vi "IsArrayConstant__slk_mt.vi"(7 "create enum configure":T1, 8 "error in (no error)":errorcluster, 11 "selection list":refnum<vi>[](array[refnum])) -> (0 "error out":errorcluster, 2 "position":cluster{"Left":i32, "Top":i32}, 3 "values":string[](array[string]), 4 "not?":bool)   [LabVIEW 2010]
uses:
  TypeDef/TypeDef_CreateEnumConfigure__slk_mt.ctl
  Library/Lazyboots Menu Tool.lvlib
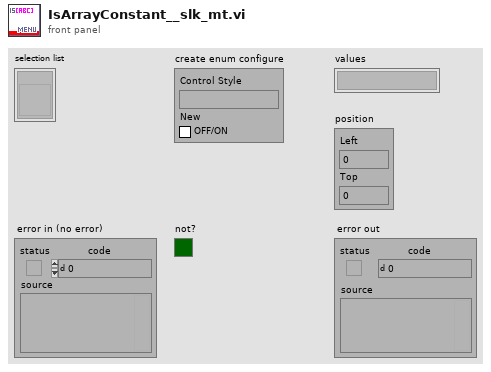
[diagram p1: front panel]
types:
  T1 = typedef "Lazyboots Menu Tool.lvlib/TypeDef_CreateEnumConfigure__slk_mt.ctl" = cluster{"Control Style":string, "New":bool}
  T2 = typedef "LVPositionTypeDef.ctl" = cluster{"Left":i32, "Top":i32}
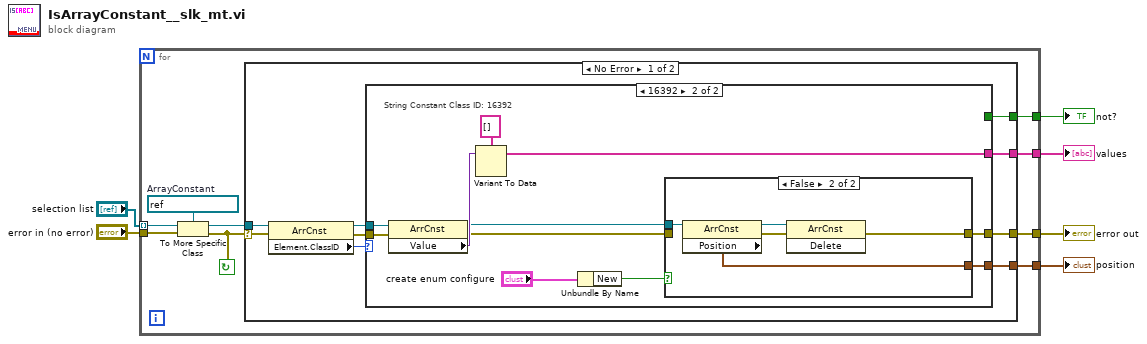
[diagram p0: block diagram]
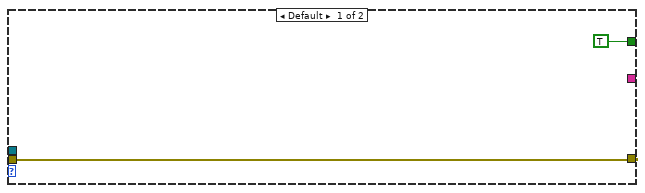
[diagram p2: hidden frame]
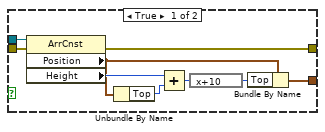
[diagram p3: hidden frame]
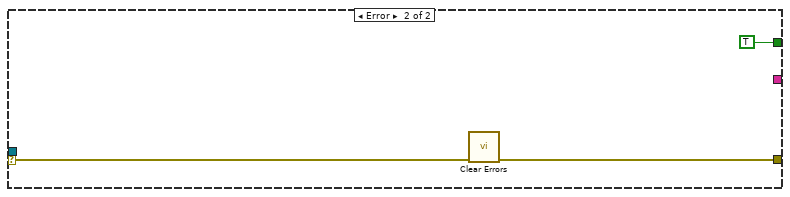
[diagram p4: hidden frame]
diagram:
  n1 = for {
    tunnel: "error in (no error)" -> [w15]
    tunnel: "selection list" -> [w13] mode=indexing
    tunnel: [w11] -> w3
    tunnel: [w9] -> w4
    tunnel: [w8] -> w2
    tunnel: [w7] -> w1
    stop <- w12 continue-if-true
    w14 = refnum<vi> refnum  # ArrayConstant
    n2 = To More Specific Class(target class=w14, reference=w13, error in=w15) -> (specific class reference=w10:refnum<vi>, error out=w12:errorcluster)
    n3 = case shown="No Error" w12 {
      selector: w12 -> [w21 w54]
      tunnel: [w18 w53] -> w11
      tunnel: w10 -> [w24 _]
      tunnel: [w23 _] -> w9
      tunnel: [w17 _] -> w8
      tunnel: [w16 TRUE] -> w7
      frame No Error {
        n4 = property class="ArrCnst"(reference=w24, error in=w21) -> (reference out=w22:refnum<vi>, error out=w20:errorcluster, "Element.ClassID"=w19:u32)
        n5 = case shown="16392" w19 {
          tunnel: [_ w33] -> w23
          tunnel: w22 -> [_ w34]
          tunnel: w20 -> [w26 w35]
          tunnel: [w26 w32] -> w18
          tunnel: [_ w29] -> w17
          tunnel: [TRUE _] -> w16
          frame Default {
          }
          frame 16392 {
            # "String Constant Class ID: 16392"
            n6 = property class="ArrCnst"(reference=w34, error in=w35) -> (reference out=w31:refnum<vi>, error out=w30:errorcluster, "Value"=w37:variant)
            n7 = Variant To Data(Variant=w37, type=string[] []) -> (data=w29:string[])  [unwired: 1 in, 1 out]
            n8 = Unbundle By Name("create enum configure") -> ("New"=w27:bool)
            n9 = case shown="False" w27 {
              tunnel: [w43 w48] -> w32
              tunnel: [w42 w51] -> w33
              tunnel: w30 -> [w39 _]
              tunnel: w31 -> [w38 w47]
              frame True {
                n10 = property class="ArrCnst"(reference=w38, error in=w39) -> (error out=w43:errorcluster, "Position"=w41:T2, "Height"=w45:u32)  [unwired: 1 out]
                n11 = Unbundle By Name(w41) -> ("Top"=w44:i32)
                n12 = Add(x=w45, y=w44) -> (x+y=w46:u32)
                n13 = expression code="x+10"(w46) -> (w40:u32)
                n14 = Bundle By Name(cluster=w41, "Top"=w40) -> (w42:T2)
              }
              frame False {
                n15 = property class="ArrCnst"(reference=w47) -> (reference out=w49:refnum<vi>, error out=w50:errorcluster, "Position"=w51:T2)  [unwired: 1 in]
                n16 = invoke class="ArrCnst" method="Delete"(reference=w49, error in=w50) -> (error out=w48:errorcluster)  [unwired: 1 in, 2 out]
              }
            }
          }
        }
      }
      frame Error {
        n17 = call <vilib>:"Clear Errors.vi"("error in (no error)"=w54) -> ("error out"=w53:errorcluster)  [unwired: 6 in]
      }
    }
  }
  "values" <- w2
  "position" <- w4
  "error out" <- w3
  "not?" <- w1
